vi "Save_waveform_settings_to_xls_Core.vi"() -> ()   [LabVIEW 2011]
uses:
  CoDiS_Velebit.llb/Types_of_analyses_Erraring.ctl
  CoDiS_Velebit.llb/Waveforms_cluster_Erraring.ctl
  CoDiS_Velebit.llb/Unit_names_Erraring.ctl
  CoDiS_Velebit.llb/Data_sources_Erraring.ctl
  CoDiS_Velebit.llb/Types_of_signals_Erraring.ctl
  CoDiS_Velebit.llb/Analysis_parameters_cluster_Erraring.ctl
  <vilib>/Analysis/3filter.llb/Filter Passband Type.ctl
  CoDiS_Velebit.llb/Integration_types_Erraring.ctl
  <vilib>/Utility/file.llb/Write To Spreadsheet File (string).vi
  <vilib>/Analysis/NI_AALBase.lvlib
panel:
  out "Analysis Parameters Cluster":T1={"DC"={"Analyze data from 1st trigger to last (if possible)? (FALSE=analyze everything)"=FALSE}, "DCExtrema"={"Calculate DC from all Pole Values"=FALSE, "Poles to use in DC calculation (if Calculate DC from all Pole Values is FALSE)"=[], "Condition Vector Label begin Part (MinPole or MaxPole)"="", "Addition to Condition Vector Label (example: 000)"=""}, "RPM"={"Signal Threshold"=0.0, "Pulse Width (should be >= 2 depending on signal noise)"=0, "Trigger on rising edge? (FALSE=trigger on falling)"=FALSE}, "Smax"={"Combine with which Waveform Label? (for example: RV001)"="", "Calculate from time-averaged signal on one revolution?"=FALSE, "Analyze data from 1st trigger to last (if possible)? (FALSE=analyze everything)"=FALSE, "Filter Parameters"={"Filter signal?"=FALSE, "filter type"=enum."Lowpass", "high cutoff freq: fh"=0.45000000000000007, "low cutoff freq: fl"=0.12500000000000006, "order"=2, "Process as ring-buffer signal?"=FALSE}, "Gliding Parameters"={"Glide signal?"=FALSE, "Number of points for gliding"=0}, "Average all calculated values for Smax - if present (each revolution)? (FALSE=take absolute maximum)"=FALSE, "Addition to Condition Vector Label (example: 000)"=""}, "SP2Pmax"={"Combine with which Waveform Label? (for example: RV001)"="", "Calculate from time-averaged signal on one revolution?"=FALSE, "Analyze data from 1st trigger to last (if possible)? (FALSE=analyze everything)"=FALSE, "Filter Parameters"={"Filter signal?"=FALSE, "filter type"=enum."Lowpass", "high cutoff freq: fh"=0.45000000000000007, "low cutoff freq: fl"=0.12500000000000006, "order"=2, "Process as ring-buffer signal?"=FALSE}, "Gliding Parameters"={"Glide signal?"=FALSE, "Number of points for gliding"=0}, "Average all calculated values for SP2Pmax - if present (each revolution)? (FALSE=take absolute maximum)"=FALSE, "Addition to Condition Vector Label (example: 000)"=""}, "snA"={"What harmonic?"=0.0, "Calculate Amplitude (TRUE) or RMS (FALSE)?"=FALSE, "Multiplication Factor"=0.0, "Calculate Amplitude for Air Gap type signals? (from MinPole Values)"=FALSE}, "snPh"={"What harmonic?"=0.0}, "Peak"={"Calculate from time-averaged signal (one-revolution)?"=FALSE, "Analyze data from 1st trigger to last (if possible)? (FALSE=analyze everything)"=FALSE, "Filter Parameters"={"Filter signal?"=FALSE, "filter type"=enum."Lowpass", "high cutoff freq: fh"=0.45000000000000007, "low cutoff freq: fl"=0.12500000000000006, "order"=2, "Process as ring-buffer signal?"=FALSE}, "Gliding Parameters"={"Glide signal?"=FALSE, "Number of points for gliding"=0}, "Average all calculated values for Peak - if present (each revolution)? (FALSE=take absolute maximum)"=FALSE, "Addition to Condition Vector Label (example: 000)"=""}, "Peak2Peak"={"Calculate from time-averaged signal (one-revolution)?"=FALSE, "Analyze data from 1st trigger to last (if possible)? (FALSE=analyze everything)"=FALSE, "Gliding Parameters"={"Glide signal?"=FALSE, "Number of points for gliding"=0}, "Filter Parameters"={"Filter signal?"=FALSE, "filter type"=enum."Lowpass", "high cutoff freq: fh"=0.45000000000000007, "low cutoff freq: fl"=0.12500000000000006, "order"=2, "Process as ring-buffer signal?"=FALSE}, "Average all calculated values for Peak2Peak - if present (each revolution)? (FALSE=take absolute maximum)"=FALSE, "Addition to Condition Vector Label (example: 000)"=""}, "EqPeak"={"Calculate from time-averaged signal (one-revolution)?"=FALSE, "Analyze data from 1st trigger to last (if possible)? (FALSE=analyze everything)"=FALSE, "Average all calculated values for EqPeak - if present (each revolution)? (FALSE=take absolute maximum)"=FALSE, "Filter Parameters"={"Filter signal?"=FALSE, "filter type"=enum."Lowpass", "high cutoff freq: fh"=0.45000000000000007, "low cutoff freq: fl"=0.12500000000000006, "order"=2, "Process as ring-buffer signal?"=FALSE}, "Which Condition Vector Label addition to use for RMS (example: 001)"="", "Addition to Condition Vector Label (example: 000)"=""}, "RMS"={"Calculate from time-averaged signal (one-revolution)?"=FALSE, "Analyze data from 1st trigger to last (if possible)? (FALSE=analyze everything)"=FALSE, "Subtract DC before RMS calculation?"=FALSE, "Filter Parameters"={"Filter signal?"=FALSE, "filter type"=enum."Lowpass", "high cutoff freq: fh"=0.45000000000000007, "low cutoff freq: fl"=0.12500000000000006, "order"=2, "Process as ring-buffer signal?"=FALSE}, "Gliding Parameters"={"Glide signal?"=FALSE, "Number of points for gliding"=0}, "Average all calculated values for RMS - if present (each revolution)? (FALSE=take absolute maximum)"=FALSE, "Addition to Condition Vector Label (example: 000)"=""}, "Rest"={"Calculate from all calculated harmonics?"=FALSE, "Condition Vector Label to use for substraction (if Calculate from all calculated harmonics?=FALSE)"=[], "Calculate by subtracting from EqPeak Value? (FALSE=calculate by subtracting from RMS Value)"=TRUE, "Which Condition Vector Label addition to use for EqPeak (example: 001)"="", "Addition to Condition Vector Label (example: 000)"=""}, "MinByPole"={"First Pole Number after Trigger (indexes correspond to Normal regime settings)"=[], "Are Pole Numbers in ascending order in time?  (indexes correspond to Normal regime settings)"=[], "Average all calculated values for that Pole? (FALSE=take absolute minimum)"=FALSE, "Coerce Upper Limit"=0.0, "Compensate 1st harmonic in waveform?"=FALSE}, "MinExtrema"={"Calculate Min Extrema from all Pole Values"=FALSE, "Poles to use in Min Extrema calculation (if Calculate Min Extrema from all Pole Values is FALSE)"=[], "Condition Vector Label begin Part (MinPole or MaxPole)"=""}, "MaxByPole"={"First Pole Number after Trigger (indexes correspond to Normal regime settings)"=[], "Are Pole Numbers in ascending order in time? (indexes correspond to Normal regime settings)"=[], "Average all calculated values for that Pole? (FALSE=take absolute maximum)"=FALSE, "Calculate with abs(Signal)?"=FALSE, "Subtract DC before calculation?"=FALSE, "Coerce Lower Limit"=0.0}, "MaxExtrema"={"Calculate Max Extrema from all Pole Values"=FALSE, "Poles to use in Max Extrema calculation (if Calculate Max Extrema from all Pole Values is FALSE)"=[], "Condition Vector Label begin Part (MinPole or MaxPole)"=""}, "MaxDiffByPole"={"First Pole Number after Trigger (indexes correspond to Normal regime settings)"=[], "Are Pole Numbers in ascending order in time? (indexes correspond to Normal regime settings)"=[], "Condition Vector Label begin Part (MinPole or MaxPole)"=""}, "Min"={"Analyze data from 1st trigger to last (if possible)? (FALSE=analyze everything)"=FALSE, "Calculate from time-averaged signal on one revolution?"=FALSE, "Gliding Parameters"={"Glide signal?"=FALSE, "Number of points for gliding"=0}, "Average all calculated values for Min - if present (each revolution)? (FALSE=take absolute maximum)"=FALSE}, "Max"={"Analyze data from 1st trigger to last (if possible)? (FALSE=analyze everything)"=FALSE, "Calculate from time-averaged signal on one revolution?"=FALSE, "Gliding Parameters"={"Glide signal?"=FALSE, "Number of points for gliding"=0}, "Average all calculated values for Max - if present (each revolution)? (FALSE=take absolute maximum)"=FALSE}, "ActivePower"={"Calculate from Phase Voltages and Currents?"=FALSE, "Phase Voltage Condition Vector Label (R, S, T) (for example: VOL000.s24.00A, VOL001.s24.00A, VOL002.s24.00A)"=[], "Phase Current Condition Vector Label (R, S, T) (for example: CURR000.s24.00A, CURR001.s24.00A, CURR002.s24.00A)"=[]}, "ReactivePower"={"Calculate from Phase Voltages and Currents?"=FALSE, "Phase Voltage Condition Vector Label (R, S, T) (for example: VOL000.s24.00A, VOL001.s24.00A, VOL002.s24.00A)"=[], "Phase Current Condition Vector Label (R, S, T) (for example: CURR000.s24.00A, CURR001.s24.00A, CURR002.s24.00A)"=[]}, "LoadAngleDelta"={"What harmonic? (for example 24th (48 pole machine))"=0.0, "Delta0"=0.0, "Which Voltage Waveform Label? (for example: VOL000)"="", "Combine (multiply) with which Air Gap Waveform Label? (for example: AG000)"="", "Multiplication Factor"=0.0}, "ActivePowerByIntegration"={"Phase Voltage Waveform Labels (R,S,T)"=[], "Phase Current Waveform Labels (R,S,T)"=[], "Analyze data from 1st trigger to last (if possible)? (FALSE=analyze everything)"=FALSE}, "RectivePowerByIntegration"={"Phase Voltage Waveform Vector Labels (R,S,T)"=[], "Phase Current Waveform Labels (R,S,T)"=[], "System Electric Frequency [Hz]"=0.0, "Analyze data from 1st trigger to last (if possible)? (FALSE=analyze everything)"=FALSE}, "Ampl@Freq"={"Frequency [Hz]"=0.0, "Calculate Amplitude? (FALSE=calculate RMS)"=FALSE}, "PhaseDifference"={"Combine with which Waveform Label?"=""}, "CosFi"={"Voltage Waveform Labels (R,S,T)"=[], "Current Waveform Labels (R,S,T)"=[]}, "Total THD"={"THD Condition Vector Label (R, S, T) (for example: VOL000.THD, VOL001.THD, VOL002.THD)"=[]}, "Crest Factor"={"Addition to Condition Vector Label (example: 000)"="", "Which Condition Vector Label addition to use for Peak (example: 001)"="", "Which Condition Vector Label addition to use for RMS (example: 001)"=""}} {"SP2Pmax"."Filter Parameters"."low cutoff freq: fl" format="%0.4f"; "SP2Pmax"."Filter Parameters"."high cutoff freq: fh" format="%0.2f"; "LoadAngleDelta"."Multiplication Factor" format="%.1f"; "LoadAngleDelta"."What harmonic? (for example 24th (48 pole machine))" format="%.1f"; "Peak2Peak"."Filter Parameters"."low cutoff freq: fl" format="%0.4f"; "Peak2Peak"."Filter Parameters"."high cutoff freq: fh" format="%0.2f"; "RMS"."Filter Parameters"."low cutoff freq: fl" format="%0.4f"; "RMS"."Filter Parameters"."high cutoff freq: fh" format="%0.2f"; "EqPeak"."Filter Parameters"."low cutoff freq: fl" format="%0.4f"; "EqPeak"."Filter Parameters"."high cutoff freq: fh" format="%0.2f"; "Peak"."Filter Parameters"."low cutoff freq: fl" format="%0.4f"; "Peak"."Filter Parameters"."high cutoff freq: fh" format="%0.2f"; "snPh"."What harmonic?" format="%.1f"; "snA"."Multiplication Factor" format="%.1f"; "snA"."What harmonic?" format="%.1f"; "Smax"."Filter Parameters"."low cutoff freq: fl" format="%0.4f"; "Smax"."Filter Parameters"."high cutoff freq: fh" format="%0.2f"; "RPM"."Signal Threshold" format="%.1f"}
  in  "Waveform Cluster DEFAULT":T3={"Configuration File loaded successfully? "=FALSE, "Is this new configuration?"=FALSE, "Unit Name"=enum."Unit 2", "Waveform Source"=[enum."Source 2", enum."Source 2", enum."Source 2", enum."Source 2", enum."Source 2", enum."Source 2", enum."Source 2", enum."Source 2", enum."Source 2", enum."Source 2", enum."Source 2", enum."Source 2", enum."Source 2", enum."Source 2", enum."Source 2", enum."Source 2", enum."Source 2", enum."Source 2", enum."Source 2", enum."Source 2", enum."Source 2", enum."Source 2", enum."Source 2", enum."Source 2", enum."Source 2", enum."Source 2"], "Use CoDiS server Timestamp (on FALSE uses Processing Unit Timestamp)?"=FALSE, "Sampling Rate [Hz]"=[2048, 2048, 2048, 2048, 2048, 2048, 2048, 2048, 2048, 2048, 2048, 2048, 2048, 2048, 2048, 2048, 2048, 2048, 2048, 2048, 2048, 2048, 2048, 2048, 2048, 2048], "Timestamp (DBL)"=0.0, "Mode of Operation - Normal"="", "Mode of Operation - Diagnostic"="", "Waveform Physical Channel"=[], "Waveform Label"=["TRG000", "TRG001", "RV000", "RV001", "RV002", "RV003", "RV004", "RV005", "RV006", "RV007", "AV000", "AV001", "AV002", "AV003", "AV004", "AV005", "AV006", "AV007", "AXD000", "AXD001", "AV008", "AV009", "AG000", "AG001", "MX000", "PROC000"], "Waveform Name"=[], "Signal Type"=[], "Is this Main Trigger Signal?"=[], "Slope"=[0.0, 0.0, 0.0, 0.0, 0.0, 0.0, 0.0, 0.0, 0.0, 0.0, 0.0, 0.0, 0.0, 0.0, 0.0, 0.0, 0.0, 0.0, 0.0, 0.0, 0.0, 0.0, 0.0, 0.0, 0.0, 0.0], "Intercept"=[], "Waveform Values"=[], "Analyse?"=[TRUE, TRUE, TRUE, TRUE, TRUE, TRUE, TRUE, TRUE, TRUE, TRUE, TRUE, TRUE, TRUE, TRUE, TRUE, TRUE, TRUE, TRUE, TRUE, TRUE, TRUE, TRUE, TRUE, TRUE, TRUE, TRUE], "Save to database?"=[], "Analyses to Perform"=[], "Perform this analysis on a CoDiS server?"=[], "General Parameters"={"Number of Poles"=0, "Grid Frequency"=0.0}, "Analysis Parameters"=[], "Save now to dBase?"=FALSE, "Waveform Length for Saving [s]"=5, "Pretrigger Length when Saving Waveform [s]"=0, "Next Timestamp to autosave at (DBL)"=0.0, "Description of Waveforms Events"="", "Event Type"="", "Save next RS event entirely? (on FALSE uses How many basic (acquisition) blocks of data (loops) to save?"=FALSE, "Regime Name for which to save next RS event entirely"="", "Integration type"=[], "Channel not OK?"=[], "Channel Not OK?  Relay Number (-1 = none, 0, ..., MAX)"=[], "Array of FPGA Filter Parameters"=[], "Pre-Alarm Delay in Number of Loops "=0, "Pre-Trip Delay in Number of Loops "=0} {"Analysis Parameters"."SP2Pmax"."Filter Parameters"."low cutoff freq: fl" format="%0.4f"; "Analysis Parameters"."SP2Pmax"."Filter Parameters"."high cutoff freq: fh" format="%0.2f"; "Analysis Parameters"."LoadAngleDelta"."Multiplication Factor" format="%.1f"; "Analysis Parameters"."LoadAngleDelta"."What harmonic? (for example 24th (48 pole machine))" format="%.1f"; "Analysis Parameters"."Peak2Peak"."Filter Parameters"."low cutoff freq: fl" format="%0.4f"; "Analysis Parameters"."Peak2Peak"."Filter Parameters"."high cutoff freq: fh" format="%0.2f"; "Analysis Parameters"."RMS"."Filter Parameters"."order" format="%0.4f"; "Analysis Parameters"."RMS"."Filter Parameters"."low cutoff freq: fl" format="%0.2f"; "Analysis Parameters"."RMS"."Filter Parameters"."high cutoff freq: fh" format="%0.2f"; "Analysis Parameters"."EqPeak"."Filter Parameters"."low cutoff freq: fl" format="%0.4f"; "Analysis Parameters"."EqPeak"."Filter Parameters"."high cutoff freq: fh" format="%0.2f"; "Analysis Parameters"."Peak"."Filter Parameters"."low cutoff freq: fl" format="%0.4f"; "Analysis Parameters"."Peak"."Filter Parameters"."high cutoff freq: fh" format="%0.2f"; "Analysis Parameters"."snPh"."What harmonic?" format="%.1f"; "Analysis Parameters"."snA"."Multiplication Factor" format="%.1f"; "Analysis Parameters"."snA"."What harmonic?" format="%.1f"; "Analysis Parameters"."Smax"."Filter Parameters"."low cutoff freq: fl" format="%0.4f"; "Analysis Parameters"."Smax"."Filter Parameters"."high cutoff freq: fh" format="%0.2f"; "Analysis Parameters"."RPM"."Signal Threshold" format="%.1f"}
  out "2D Array of Names Values IN":string[][](array[string])
  out "TempAnalysis":T7
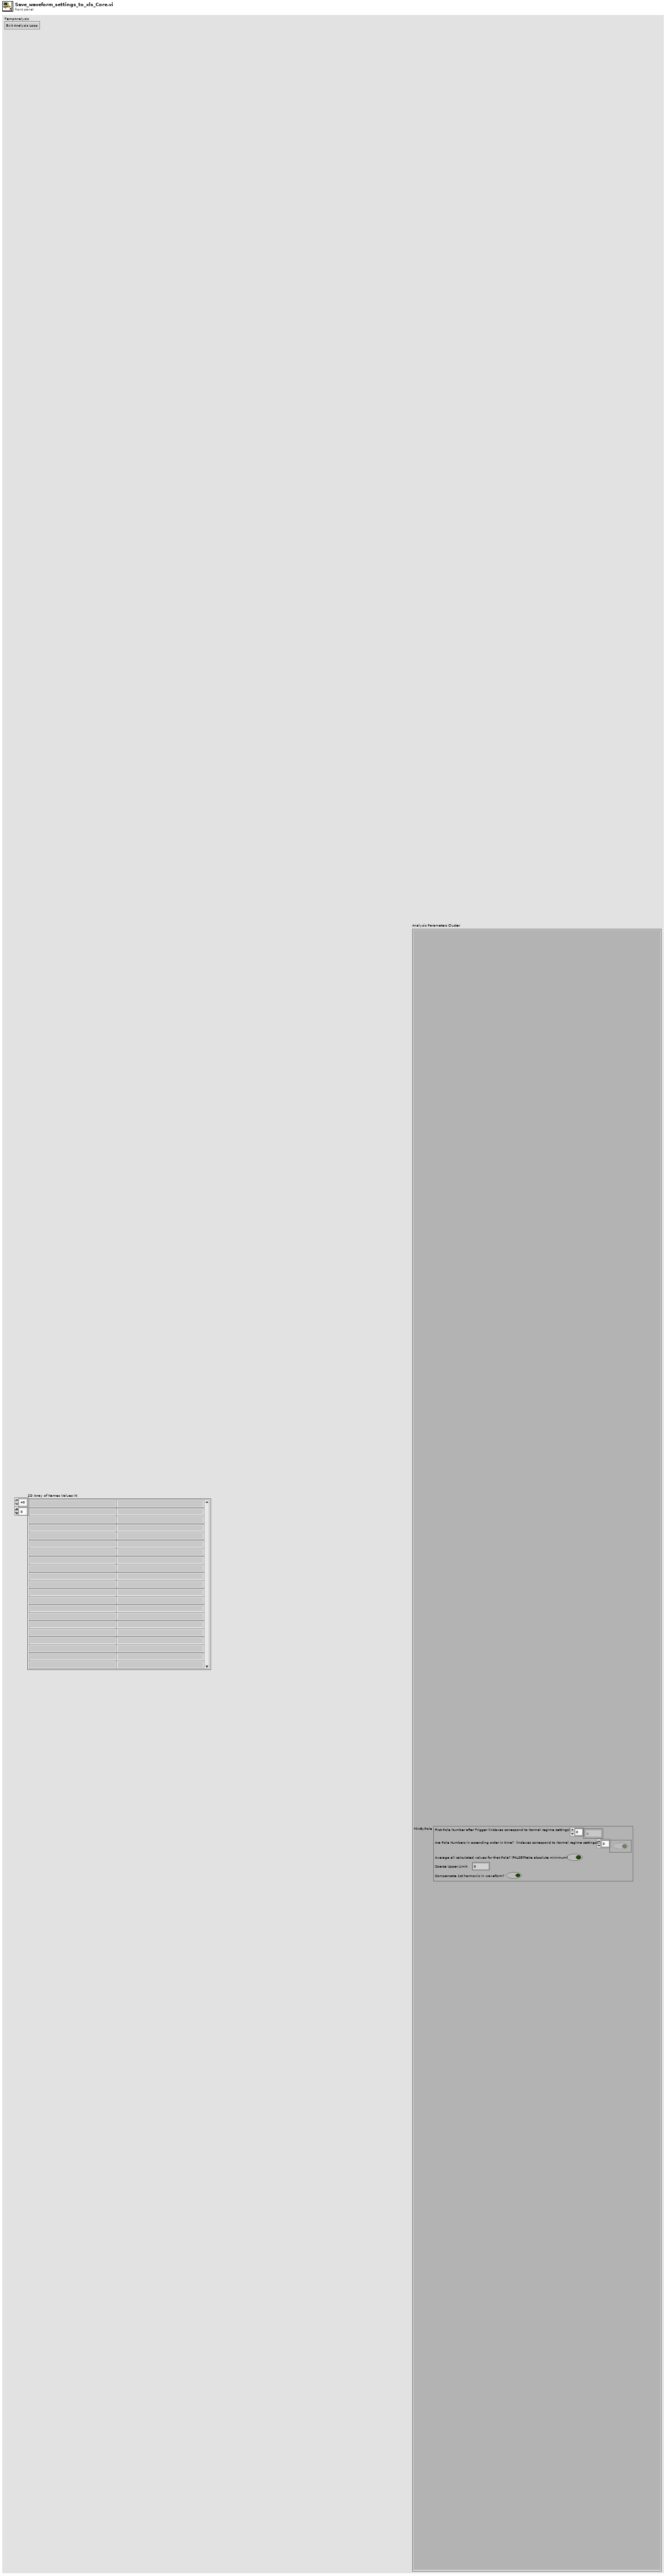
[diagram p1: front panel]
types:
  T1 = typedef "Analysis_parameters_cluster_Erraring.ctl" = cluster{"DC":cluster{"Analyze data from 1st trigger to last (if possible)? (FALSE=analyze everything)":bool}, "DCExtrema":cluster{"Calculate DC from all Pole Values":bool, "Poles to use in DC calculation (if Calculate DC from all Pole Values is FALSE)":u8[], "Condition Vector Label begin Part (MinPole or MaxPole)":string, "Addition to Condition Vector Label (example: 000)":string}, "RPM":cluster{"Signal Threshold":sgl, "Pulse Width (should be >= 2 depending on signal noise)":i32, "Trigger on rising edge? (FALSE=trigger on falling)":bool}, "Smax":cluster{"Combine with which Waveform Label? (for example: RV001)":string, "Calculate from time-averaged signal on one revolution?":bool, "Analyze data from 1st trigger to last (if possible)? (FALSE=analyze everything)":bool, "Filter Parameters":cluster{"Filter signal?":bool, "filter type":T2, "high cutoff freq: fh":dbl, "low cutoff freq: fl":dbl, "order":i32, "Process as ring-buffer signal?":bool}, "Gliding Parameters":cluster{"Glide signal?":bool, "Number of points for gliding":u16}, "Average all calculated values for Smax - if present (each revolution)? (FALSE=take absolute maximum)":bool, "Addition to Condition Vector Label (example: 000)":string}, "SP2Pmax":cluster{"Combine with which Waveform Label? (for example: RV001)":string, "Calculate from time-averaged signal on one revolution?":bool, "Analyze data from 1st trigger to last (if possible)? (FALSE=analyze everything)":bool, "Filter Parameters":cluster{"Filter signal?":bool, "filter type":T2, "high cutoff freq: fh":dbl, "low cutoff freq: fl":dbl, "order":i32, "Process as ring-buffer signal?":bool}, "Gliding Parameters":cluster{"Glide signal?":bool, "Number of points for gliding":u16}, "Average all calculated values for SP2Pmax - if present (each revolution)? (FALSE=take absolute maximum)":bool, "Addition to Condition Vector Label (example: 000)":string}, "snA":cluster{"What harmonic?":sgl, "Calculate Amplitude (TRUE) or RMS (FALSE)?":bool, "Multiplication Factor":sgl, "Calculate Amplitude for Air Gap type signals? (from MinPole Values)":bool}, "snPh":cluster{"What harmonic?":sgl}, "Peak":cluster{"Calculate from time-averaged signal (one-revolution)?":bool, "Analyze data from 1st trigger to last (if possible)? (FALSE=analyze everything)":bool, "Filter Parameters":cluster{"Filter signal?":bool, "filter type":T2, "high cutoff freq: fh":dbl, "low cutoff freq: fl":dbl, "order":i32, "Process as ring-buffer signal?":bool}, "Gliding Parameters":cluster{"Glide signal?":bool, "Number of points for gliding":u16}, "Average all calculated values for Peak - if present (each revolution)? (FALSE=take absolute maximum)":bool, "Addition to Condition Vector Label (example: 000)":string}, "Peak2Peak":cluster{"Calculate from time-averaged signal (one-revolution)?":bool, "Analyze data from 1st trigger to last (if possible)? (FALSE=analyze everything)":bool, "Gliding Parameters":cluster{"Glide signal?":bool, "Number of points for gliding":u16}, "Filter Parameters":cluster{"Filter signal?":bool, "filter type":T2, "high cutoff freq: fh":dbl, "low cutoff freq: fl":dbl, "order":i32, "Process as ring-buffer signal?":bool}, "Average all calculated values for Peak2Peak - if present (each revolution)? (FALSE=take absolute maximum)":bool, "Addition to Condition Vector Label (example: 000)":string}, "EqPeak":cluster{"Calculate from time-averaged signal (one-revolution)?":bool, "Analyze data from 1st trigger to last (if possible)? (FALSE=analyze everything)":bool, "Average all calculated values for EqPeak - if present (each revolution)? (FALSE=take absolute maximum)":bool, "Filter Parameters":cluster{"Filter signal?":bool, "filter type":T2, "high cutoff freq: fh":dbl, "low cutoff freq: fl":dbl, "order":i32, "Process as ring-buffer signal?":bool}, "Which Condition Vector Label addition to use for RMS (example: 001)":string, "Addition to Condition Vector Label (example: 000)":string}, "RMS":cluster{"Calculate from time-averaged signal (one-revolution)?":bool, "Analyze data from 1st trigger to last (if possible)? (FALSE=analyze everything)":bool, "Subtract DC before RMS calculation?":bool, "Filter Parameters":cluster{"Filter signal?":bool, "filter type":T2, "high cutoff freq: fh":dbl, "low cutoff freq: fl":dbl, "order":i32, "Process as ring-buffer signal?":bool}, "Gliding Parameters":cluster{"Glide signal?":bool, "Number of points for gliding":u16}, "Average all calculated values for RMS - if present (each revolution)? (FALSE=take absolute maximum)":bool, "Addition to Condition Vector Label (example: 000)":string}, "Rest":cluster{"Calculate from all calculated harmonics?":bool, "Condition Vector Label to use for substraction (if Calculate from all calculated harmonics?=FALSE)":string[], "Calculate by subtracting from EqPeak Value? (FALSE=calculate by subtracting from RMS Value)":bool, "Which Condition Vector Label addition to use for EqPeak (example: 001)":string, "Addition to Condition Vector Label (example: 000)":string}, "MinByPole":cluster{"First Pole Number after Trigger (indexes correspond to Normal regime settings)":u8[], "Are Pole Numbers in ascending order in time?  (indexes correspond to Normal regime settings)":bool[], "Average all calculated values for that Pole? (FALSE=take absolute minimum)":bool, "Coerce Upper Limit":sgl, "Compensate 1st harmonic in waveform?":bool}, "MinExtrema":cluster{"Calculate Min Extrema from all Pole Values":bool, "Poles to use in Min Extrema calculation (if Calculate Min Extrema from all Pole Values is FALSE)":u8[], "Condition Vector Label begin Part (MinPole or MaxPole)":string}, "MaxByPole":cluster{"First Pole Number after Trigger (indexes correspond to Normal regime settings)":u8[], "Are Pole Numbers in ascending order in time? (indexes correspond to Normal regime settings)":bool[], "Average all calculated values for that Pole? (FALSE=take absolute maximum)":bool, "Calculate with abs(Signal)?":bool, "Subtract DC before calculation?":bool, "Coerce Lower Limit":sgl}, "MaxExtrema":cluster{"Calculate Max Extrema from all Pole Values":bool, "Poles to use in Max Extrema calculation (if Calculate Max Extrema from all Pole Values is FALSE)":u8[], "Condition Vector Label begin Part (MinPole or MaxPole)":string}, "MaxDiffByPole":cluster{"First Pole Number after Trigger (indexes correspond to Normal regime settings)":u8[], "Are Pole Numbers in ascending order in time? (indexes correspond to Normal regime settings)":bool[], "Condition Vector Label begin Part (MinPole or MaxPole)":string}, "Min":cluster{"Analyze data from 1st trigger to last (if possible)? (FALSE=analyze everything)":bool, "Calculate from time-averaged signal on one revolution?":bool, "Gliding Parameters":cluster{"Glide signal?":bool, "Number of points for gliding":u16}, "Average all calculated values for Min - if present (each revolution)? (FALSE=take absolute maximum)":bool}, "Max":cluster{"Analyze data from 1st trigger to last (if possible)? (FALSE=analyze everything)":bool, "Calculate from time-averaged signal on one revolution?":bool, "Gliding Parameters":cluster{"Glide signal?":bool, "Number of points for gliding":u16}, "Average all calculated values for Max - if present (each revolution)? (FALSE=take absolute maximum)":bool}, "ActivePower":cluster{"Calculate from Phase Voltages and Currents?":bool, "Phase Voltage Condition Vector Label (R, S, T) (for example: VOL000.s24.00A, VOL001.s24.00A, VOL002.s24.00A)":string[], "Phase Current Condition Vector Label (R, S, T) (for example: CURR000.s24.00A, CURR001.s24.00A, CURR002.s24.00A)":string[]}, "ReactivePower":cluster{"Calculate from Phase Voltages and Currents?":bool, "Phase Voltage Condition Vector Label (R, S, T) (for example: VOL000.s24.00A, VOL001.s24.00A, VOL002.s24.00A)":string[], "Phase Current Condition Vector Label (R, S, T) (for example: CURR000.s24.00A, CURR001.s24.00A, CURR002.s24.00A)":string[]}, "LoadAngleDelta":cluster{"What harmonic? (for example 24th (48 pole machine))":sgl, "Delta0":sgl, "Which Voltage Waveform Label? (for example: VOL000)":string, "Combine (multiply) with which Air Gap Waveform Label? (for example: AG000)":string, "Multiplication Factor":sgl}, "ActivePowerByIntegration":cluster{"Phase Voltage Waveform Labels (R,S,T)":string[], "Phase Current Waveform Labels (R,S,T)":string[], "Analyze data from 1st trigger to last (if possible)? (FALSE=analyze everything)":bool}, "RectivePowerByIntegration":cluster{"Phase Voltage Waveform Vector Labels (R,S,T)":string[], "Phase Current Waveform Labels (R,S,T)":string[], "System Electric Frequency [Hz]":sgl, "Analyze data from 1st trigger to last (if possible)? (FALSE=analyze everything)":bool}, "Ampl@Freq":cluster{"Frequency [Hz]":sgl, "Calculate Amplitude? (FALSE=calculate RMS)":bool}, "PhaseDifference":cluster{"Combine with which Waveform Label?":string}, "CosFi":cluster{"Voltage Waveform Labels (R,S,T)":string[], "Current Waveform Labels (R,S,T)":string[]}, "Total THD":cluster{"THD Condition Vector Label (R, S, T) (for example: VOL000.THD, VOL001.THD, VOL002.THD)":string[]}, "Crest Factor":cluster{"Addition to Condition Vector Label (example: 000)":string, "Which Condition Vector Label addition to use for Peak (example: 001)":string, "Which Condition Vector Label addition to use for RMS (example: 001)":string}}
  T2 = typedef "NI_AALBase.lvlib/Filter Passband Type.ctl" = enum32{"Lowpass", "Highpass", "Bandpass", "Bandstop"}
  T3 = typedef "Waveforms_cluster_Erraring.ctl" = cluster{"Configuration File loaded successfully? ":bool, "Is this new configuration?":bool, "Unit Name":T4, "Waveform Source":T5[], "Use CoDiS server Timestamp (on FALSE uses Processing Unit Timestamp)?":bool, "Sampling Rate [Hz]":u32[], "Timestamp (DBL)":dbl, "Mode of Operation - Normal":string, "Mode of Operation - Diagnostic":string, "Waveform Physical Channel":u16[], "Waveform Label":string[], "Waveform Name":string[], "Signal Type":cluster{"Signal Type":T6, "# of signal of particular type":u8}[], "Is this Main Trigger Signal?":bool[], "Slope":dbl[], "Intercept":dbl[], "Waveform Values":sgl[][], "Analyse?":bool[], "Save to database?":bool[], "Analyses to Perform":T7[][], "Perform this analysis on a CoDiS server?":bool[][], "General Parameters":cluster{"Number of Poles":u8, "Grid Frequency":sgl}, "Analysis Parameters":T1[][], "Save now to dBase?":bool, "Waveform Length for Saving [s]":u16, "Pretrigger Length when Saving Waveform [s]":u16, "Next Timestamp to autosave at (DBL)":dbl, "Description of Waveforms Events":string, "Event Type":string, "Save next RS event entirely? (on FALSE uses How many basic (acquisition) blocks of data (loops) to save?":bool, "Regime Name for which to save next RS event entirely":string, "Integration type":T8[], "Channel not OK?":bool[], "Channel Not OK?  Relay Number (-1 = none, 0, ..., MAX)":i16[], "Array of FPGA Filter Parameters":cluster{"Filter signal?":bool, "filter type":T2, "high cutoff freq: fh":dbl, "low cutoff freq: fl":dbl, "order":i32}[][], "Pre-Alarm Delay in Number of Loops ":u16, "Pre-Trip Delay in Number of Loops ":u16}
  T4 = typedef "Unit_names_Erraring.ctl" = enum16{"Not used", "Unit 1", "Unit 2", "Unit 3", "Unit 4", "Unit 5", "Unit 6", "Unit 7", "Unit 8", "Unit 9"}
  T5 = typedef "Data_sources_Erraring.ctl" = enum16{"Not Used", "Source 0", "Source 1", "Source 2", "Source 3", "Source 4", "Source 5", "Source 6", "Source 7", "Source 8", "Source 9", "Source 10", "Source 11", "Source 12", "Source 13", "Source 14", "Source 15", "Source 16", "Source 17", "Source 18", "Source 19", "Source 20"}
  T6 = typedef "Types_of_signals_Erraring.ctl" = enum16{"Not Used", "Trigger (TRG???)", "Relative Vibrations (RV???)", "Absolute Vibrations (AV???)", "Air Gap (AG???)", "Magnetic Field (MX???)", "Voltage (VOL???)", "Current (CURR???)", "Process (PROC???)", "Cavitation (CAV???)", "Non Standard (NONST???)", "Axial Displacement (AXD???)", "Absolute Vibrations Stator Core (AVSC???)"}
  T7 = typedef "Types_of_analyses_Erraring.ctl" = enum16{"Exit Analysis Loop", "Do Nothing", "RPM", "Smax", "SP2Pmax", "snA", "snPh", "Rest", "Peak", "EqPeak", "Peak2Peak", "RMS", "DC", "DC from Extrema", "Min Value", "Max Value", "Min Value by Pole", "Max Value by Pole", "Max Diff by Pole", "Max Diff Pole Number", "Min from Extrema", "Max from Extrema", "Active Power from DFT", "Active Power by Integration", "Reactive Power from DFT", "Reactive Power by Integration", "Apparent Power", "Ampl@Freq", "Phase Difference", "Load Angle Delta", "THD", "Signal Frequency", "Eta", "Non standard (CoDiS server - manual) 0", "Non standard (CoDiS server - manual) 1", "Non standard (CoDiS server - manual) 2", "Non standard (CoDiS server - manual) 3", "Non standard (CoDiS server - manual) 4", "Non standard (CoDiS server - manual) 5", "Non standard (CoDiS server - manual) 6", "Non standard (CoDiS server - manual) 7", "Non standard (CoDiS server - manual) 8", "Non standard (CoDiS server - manual) 9", "Non standard (CoDiS server - manual) 10", "Non standard (CoDiS server - manual) 11", "Non standard (CoDiS server - manual) 12", "Non standard (CoDiS server - manual) 13", "Non standard (CoDiS server - manual) 14", "Non standard (CoDiS server - manual) 15", "Non standard (CoDiS server - manual) 16", "Non standard (CoDiS server - manual) 17", "Non standard (CoDiS server - manual) 18", "Non standard (CoDiS server - manual) 19", "CosFi", "Total THD", "Crest Factor"}
  T8 = typedef "Integration_types_Erraring.ctl" = enum16{"Do not integrate", "Integrate once", "Integrate twice"}
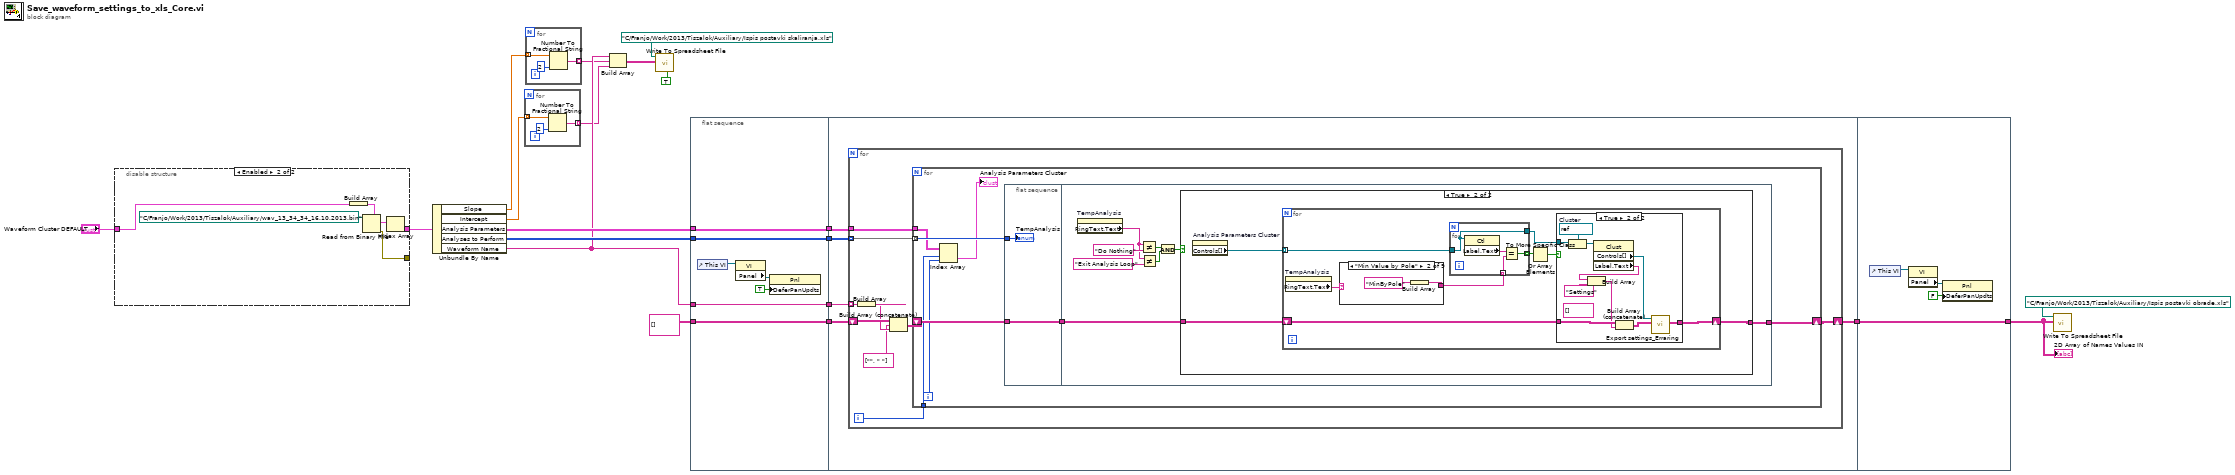
[diagram p0: block diagram]
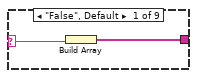
[diagram p5: hidden frame]
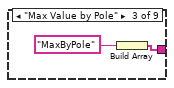
[diagram p6: hidden frame]
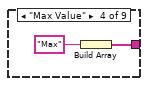
[diagram p7: hidden frame]
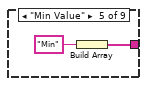
[diagram p8: hidden frame]
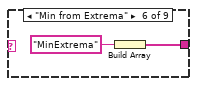
[diagram p9: hidden frame]
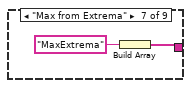
[diagram p10: hidden frame]
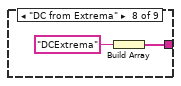
[diagram p11: hidden frame]
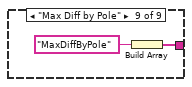
[diagram p12: hidden frame]
diagram:
  n1 = disable-structure shown="Enabled" {
    disable-tunnel: [w21 w23] -> w2
    disable-tunnel: "Waveform Cluster DEFAULT" -> [w21 w26]
    disable-tunnel: [_ w22] -> _
    frame Disabled {
    }
    frame Enabled {
      n2 = Build Array(w26) -> (w25:T3[])
      n3 = Read from Binary File(5:w25, 11:path "C:/Franjo/Work/2013/Tiszalok/Auxiliary/wav_13_34_34_16.10.2013.bin" ("file (use dialog)")) -> (0:w22:errorcluster, 2:w24:T3[])  [unwired: 4 in, 2 out]
      n4 = Index Array(array=w24) -> (element=w23:T3)  [unwired: 1 in]
    }
  }
  n5 = Unbundle By Name(w2) -> ("Slope"=w10:dbl[], "Intercept"=w9:dbl[], "Analysis Parameters"=w13:T1[][], "Analyses to Perform"=w20:T7[][], "Waveform Name"=w8:string[])
  n6 = for {
    tunnel: w9 -> [w29] mode=indexing
    tunnel: [w28] -> w6 mode=indexing
    n7 = Number To Fractional String(number=w29, precision (6)=i16 2) -> (F-format string=w28:string)  [unwired: 2 in]
  }
  n8 = for {
    tunnel: w10 -> [w32] mode=indexing
    tunnel: [w31] -> w7 mode=indexing
    n9 = Number To Fractional String(number=w32, precision (6)=i16 2) -> (F-format string=w31:string)  [unwired: 2 in]
  }
  n10 = Build Array(w8, w7, w6) -> (w4:string[][])
  n11 = call-poly <vilib>:"Write To Spreadsheet File.vi"("transpose? (no:F)"=TRUE, "2D data"=w4, "file path (dialog if empty)"=path "C:/Franjo/Work/2013/Tiszalok/Auxiliary/Ispis postavki skaliranja.xls") -> ()  [unwired: 5 in, 1 out]
  n12 = flat-sequence {
    tunnel: string[][] [] ("2D Array of Names Values IN") -> [w39]
    tunnel: w20 -> [w40]
    tunnel: [w40] -> w17
    tunnel: [w39] -> w16
    tunnel: [w35] -> w15
    tunnel: w8 -> [w35]
    tunnel: [w34] -> w14
    tunnel: w13 -> [w34]
    tunnel: [w43] -> w18
    tunnel: w17 -> [w45]
    tunnel: w16 -> [w44]
    tunnel: w15 -> [w42]
    tunnel: w14 -> [w41]
    tunnel: [w121] -> w11
    tunnel: w18 -> [w121]
    frame #0 {
      n13 = control-ref of="This VI"() -> (w38:refnum<vi>)
      n14 = property class="VI"(reference=w38) -> ("Panel"=w37:refnum<vi>)  [unwired: 1 in, 2 out]
      n15 = property class="Pnl"(reference=w37, "DeferPanUpdts"=TRUE ("Defer Panel Updates")) -> ()  [unwired: 1 in, 2 out]
    }
    frame #1 {
      n16 = for {
        tunnel: w45 -> [w54] mode=indexing
        shift-right: [w53] -> w43
        shift-left: w44 -> [w51]
        tunnel: w42 -> [w52] mode=indexing
        tunnel: w41 -> [w47]
        i -> [w46]
        n17 = Build Array(w52) -> (w49:string[])
        n18 = Build Array (concatenate)(w51, string[] ["", " "] ("appended array"), w49) -> (w50:string[][])
        n19 = for {
          tunnel: w54 -> [w62] mode=indexing
          shift-right: [w59] -> w53
          shift-left: w50 -> [w60]
          tunnel: w47 -> [w58]
          tunnel: w46 -> [w57]
          i -> [w56]
          n20 = Index Array(array=w58, index (row)=w57, index (col)=w56) -> (element=→"Analysis Parameters Cluster":T1)
          n21 = flat-sequence {
            tunnel: w62 -> [w64]
            tunnel: [w63] -> w61
            tunnel: w60 -> [w63]
            tunnel: w61 -> [w72]
            tunnel: [w71] -> w59
            frame #0 {
              "TempAnalysis" <- w64
            }
            frame #1 {
              n22 = property on="TempAnalysis" class="Enum (strict)"() -> ("RingText.Text"=w66:string)  [unwired: 2 in, 2 out]
              n23 = Not Equal?(x=w66, y="Do Nothing") -> (x != y?=w68:bool)
              n24 = Not Equal?(x=w66, y="Exit Analysis Loop") -> (x != y?=w67:bool)
              n25 = And(x=w68, y=w67) -> (x .and. y?=w65:bool)
              n26 = case shown="True" w65 {
                tunnel: w72 -> [w73 w76]
                tunnel: [w73 w75] -> w71
                frame False {
                }
                frame True {
                  n27 = property on="Analysis Parameters Cluster" class="Clust (strict)"() -> ("Controls[]"=w74:refnum<vi>[])  [unwired: 2 in, 2 out]
                  n28 = for {
                    tunnel: w74 -> [w84] mode=indexing
                    shift-right: [w81] -> w75
                    shift-left: w76 -> [w80]
                    n29 = property on="TempAnalysis" class="Enum (strict)"() -> ("RingText.Text"=w79:string)  [unwired: 2 in, 2 out]
                    n30 = case shown="\"Min Value by Pole\"" w79 {
                      selector: w79 -> [w101 _ _ _ _ _ _ _ _]
                      tunnel: [w100 w102 w104 w106 w108 w110 w112 w114 w116] -> w83
                      frame "False", Default {
                        n31 = Build Array(w101) -> (w100:string[])
                      }
                      frame "Min Value by Pole" {
                        n32 = Build Array("MinByPole" ("y")) -> (w102:string[])
                      }
                      frame "Max Value by Pole" {
                        n33 = Build Array("MaxByPole" ("y")) -> (w104:string[])
                      }
                      frame "Max Value" {
                        n34 = Build Array("Max" ("y")) -> (w106:string[])
                      }
                      frame "Min Value" {
                        n35 = Build Array("Min" ("y")) -> (w108:string[])
                      }
                      frame "Min from Extrema" {
                        n36 = Build Array("MinExtrema" ("y")) -> (w110:string[])
                      }
                      frame "Max from Extrema" {
                        n37 = Build Array("MaxExtrema" ("y")) -> (w112:string[])
                      }
                      frame "DC from Extrema" {
                        n38 = Build Array("DCExtrema" ("y")) -> (w114:string[])
                      }
                      frame "Max Diff by Pole" {
                        n39 = Build Array("MaxDiffByPole" ("y")) -> (w116:string[])
                      }
                    }
                    n40 = for {
                      tunnel: w84 -> [w97]
                      tunnel: w83 -> [w98] mode=indexing
                      tunnel: [w97] -> w77
                      tunnel: [w96] -> w82 mode=indexing
                      n41 = property on="Property Node" class="Ctl"(reference=w97) -> ("Label.Text"=w99:string)  [unwired: 1 in, 2 out]
                      n42 = Equal?(x=w99, y=w98) -> (x = y?=w96:bool)
                    }
                    n43 = Or Array Elements(Boolean array=w82) -> (logical OR=w78:bool)
                    n44 = case shown="True" w78 {
                      tunnel: w77 -> [_ w94]
                      tunnel: [w85 w91] -> w81
                      tunnel: w80 -> [w85 w88]
                      frame False {
                      }
                      frame True {
                        (unwired) string[] [] ("appended array")
                        w95 = refnum<vi> refnum  # Cluster
                        n45 = To More Specific Class(target class=w95, reference=w94) -> (specific class reference=w93:refnum<vi>)  [unwired: 1 in, 1 out]
                        n46 = property on="Property Node" class="Clust"(reference=w93) -> ("Controls[]"=w92:refnum<vi>[], "Label.Text"=w90:string)  [unwired: 1 in, 2 out]
                        n47 = Build Array(w90, "Settings" ("element")) -> (w86:string[])
                        n48 = Build Array (concatenate)(w88, w86) -> (w87:string[][])
                        n49 = call "Export settings_Erraring.vi"("2D Array of Names Values IN"=w87, "Controls[]"=w92) -> ("2D Array of Names Values OUT"=w91:string[][])  [unwired: 9 in]
                      }
                    }
                  }
                }
              }
            }
          }
        }
      }
    }
    frame #2 {
      n50 = control-ref of="This VI"() -> (w120:refnum<vi>)
      n51 = property class="VI"(reference=w120) -> ("Panel"=w119:refnum<vi>)  [unwired: 1 in, 2 out]
      n52 = property class="Pnl"(reference=w119, "DeferPanUpdts"=FALSE ("Defer Panel Updates")) -> ()  [unwired: 1 in, 2 out]
    }
  }
  n53 = call-poly <vilib>:"Write To Spreadsheet File.vi"("2D data"=w11, "file path (dialog if empty)"=path "C:/Franjo/Work/2013/Tiszalok/Auxiliary/Ispis postavki obrade.xls") -> ()  [unwired: 6 in, 1 out]
  "2D Array of Names Values IN" <- w11
